vi "ChicagoStylePepperoniPizzaParamsStack.vi"(8 "error iN":errorcluster) -> (0 "error out":errorcluster, 2 "HierarchyParams":variant[](array[variant]), 3 "ChicagoStylePepperoniPizza":refnum<class "ChicagoStylePepperoniPizza.lvclass">)   [LabVIEW 2020, in "FactoryMethod.lvlib" / "PizzaFactoryMethod.lvlib" / "ChicagoStylePepperoniPizza.lvclass"]
uses:
  ChicagoStylePepperoniPizza.lvclass
  E:/Francesco/GitHub/Design-Patterns-GoF_-_NI-LV/Creational/FactoryMethod/Head-First_Example/PizzaFactoryMethod/Pizza/Pizza.lvclass
  Pizza/Protected/property/Read PizzaParams.vi
  ChicagoStylePepperoniPizza.lvclass/ChicagoStylePepperoniPizza.ctl
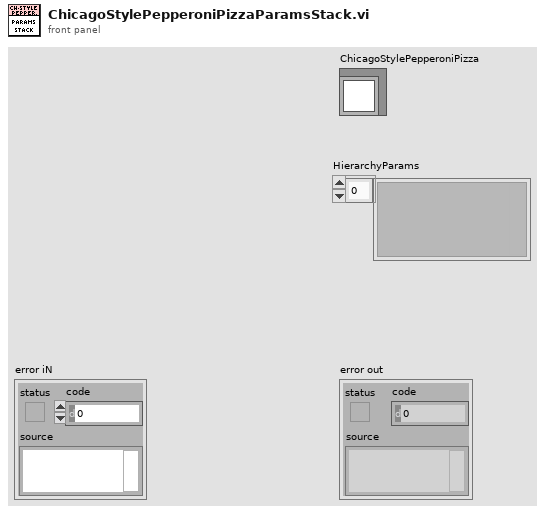
[diagram p1: front panel]
types:
  T1 = typedef "FactoryMethod.lvlib/PizzaFactoryMethod.lvlib/Pizza.lvclass/PizzaParams.ctl" = cluster{"name":string, "dough":string, "sauce":string, "toppings":string[]}
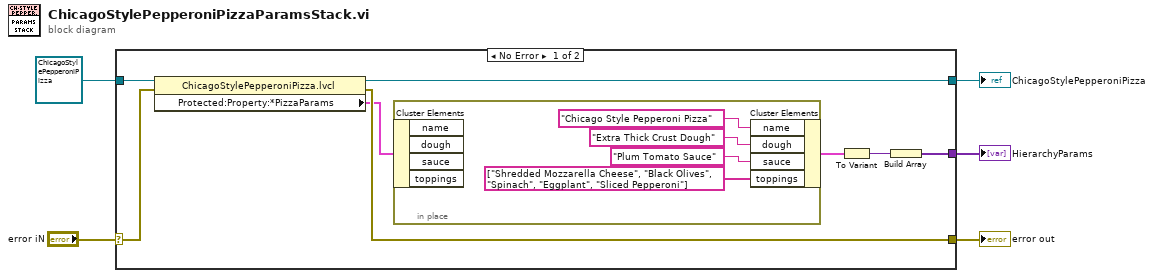
[diagram p0: block diagram]
diagram:
  n1 = case shown="No Error" "error iN" {
    selector: "error iN" -> [w13 w19]
    tunnel: [w10 w19] -> w4
    tunnel: refnum<class "ChicagoStylePepperoniPizza.lvclass"> refnum ("ChicagoStyleClamPizza") -> [w12 w18]
    tunnel: [w11 w18] -> w1
    tunnel: [w9 _] -> w3
    frame No Error {
      n2 = property class="ChicagoStylePepperoniPizza.lvcl"(reference=w12, error in=w13) -> (reference out=w11:refnum<class "ChicagoStylePepperoniPizza.lvclass">, error out=w10:errorcluster, "Protected:Property:*PizzaParams"=w7:T1)
      n3 = in-place {
        n4 = in-place-cluster #1(w7) -> ()  [unwired: 4 out]
        n5 = in-place-cluster #1("name"="Chicago Style Pepperoni Pizza", "dough"="Extra Thick Crust Dough" ("name"), "sauce"="Plum Tomato Sauce" ("name"), "toppings"=string[] ["Shredded Mozzarella Cheese", "Black Olives", "Spinach", "Eggplant", "Sliced Pepperoni"]) -> (w6:T1)
      }
      n6 = To Variant(anything=w6) -> (Variant=w8:variant)
      n7 = Build Array(w8) -> (w9:variant[])
    }
    frame Error {
    }
  }
  "error out" <- w4
  "HierarchyParams" <- w3
  "ChicagoStylePepperoniPizza" <- w1
